vi "Digitizer Scan Trigger Get Time Stamp.vi"(7 "ValBufferSize":i32=2048, 8 "error in (no error)":errorcluster {"code" format="%.0x"}, 9 "Channel":string, 10 "Record":i32 format="%.0g", 11 "instrument handle":refnum<k15>) -> (0 "error out":errorcluster {"code" format="%.0x"}, 2 "Val":string, 3 "instrument handle out":refnum<k15>)   [LabVIEW 2020, in "Keysight DAQ970.lvlib"]
doc: "Returns the trigger's time stamp of the specified reading record for digitizer module digitizing on the specified channel."
uses:
  Keysight DAQ970.lvlib
  KtDAQ970.dll
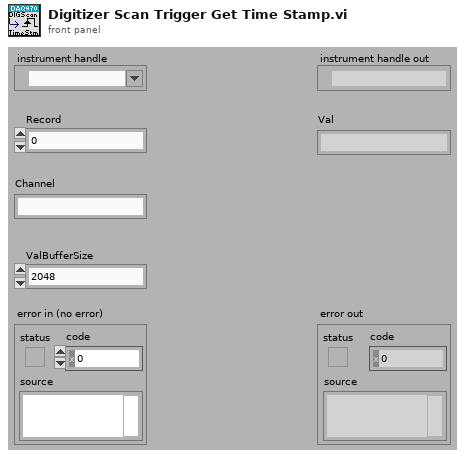
[diagram p1: front panel]
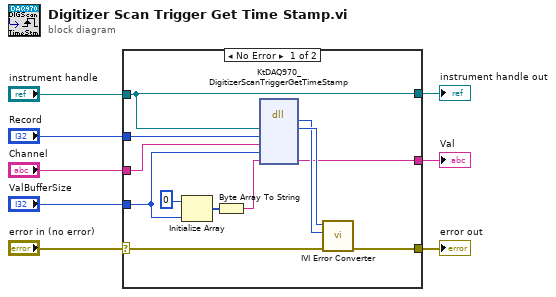
[diagram p0: block diagram]
diagram:
  n1 = case shown="No Error" "error in (no error)" {
    selector: "error in (no error)" -> [w18 w22]
    tunnel: [w17 w22] -> w8
    tunnel: "instrument handle" -> [w10 w21]
    tunnel: "Record" -> [w16 _]
    tunnel: "Channel" -> [w15 _]
    tunnel: "ValBufferSize" -> [w9 _]
    tunnel: [w11 _] -> w2
    tunnel: [w10 w21] -> w1
    frame No Error {
      n2 = Initialize Array(u8 0 ("element"), w9) -> (w13:u8[])
      n3 = Byte Array To String(unsigned byte array=w13) -> (string=w14:string)
      n4 = dll-call lib="KtDAQ970**.dll" fn="KtDAQ970_DigitizerScanTriggerGetTimeStamp"("Vi"=w10, "Record"=w16, "Channel"=w15, "ValBufferSize"=w9, "Val"=w14) -> (w19:i32, "Vi"=w20:u32, "Val"=w11:string)  [unwired: 6 in, 2 out]
      n5 = call "IVI Error Converter.vi"("error in (no error)"=w18, "IVI error code (0)"=w19, "instrument handle"=w20) -> ("error out"=w17:errorcluster)  [unwired: 7 in, 1 out]
    }
    frame Error {
    }
  }
  "error out" <- w8
  "instrument handle out" <- w1
  "Val" <- w2
